vi "test-linear-system-loop-02.vi"() -> (3 "TEst Passed":bool)   [LabVIEW 2019]
uses:
  <vilib>/Rock Robotics/WPI/ThirdParty/JAS_Junk/TrajLib/LINEAR_SYSTEM_LOOP.ctl
  <vilib>/Rock Robotics/WPI/ThirdParty/JAS_Junk/TrajLib/LINEAR_QUADRATIC_REGULATOR.ctl
  <vilib>/Analysis/Matrix/Datatypes/RealMatrix.ctl
  <vilib>/Rock Robotics/WPI/ThirdParty/JAS_Junk/TrajLib/LINEAR_PLANT_INV_FF.ctl
  <vilib>/Rock Robotics/WPI/ThirdParty/JAS_Junk/TrajLib/KALMAN_FILTER.ctl
  <vilib>/Rock Robotics/WPI/ThirdParty/JAS_Junk/TrajLib/LINEAR_SYSTEM.ctl
  <vilib>/Rock Robotics/WPI/ThirdParty/JAS_Junk/TrajLib/DCMOTOR_TYPES_ENUM.ctl
  <vilib>/Rock Robotics/WPI/ThirdParty/JAS_Junk/TrajLib/MatBuilder_Create.vi
  <vilib>/Rock Robotics/WPI/ThirdParty/JAS_Junk/TrajLib/DCMotor_GetCIM.vi
  <vilib>/Rock Robotics/WPI/ThirdParty/JAS_Junk/TrajLib/DCMotor_GetAndymark9015.vi
  <vilib>/Rock Robotics/WPI/ThirdParty/JAS_Junk/TrajLib/DCMotor_GetAndymarkRs775_125.vi
  <vilib>/Rock Robotics/WPI/ThirdParty/JAS_Junk/TrajLib/DCMotor_GetBag.vi
  <vilib>/Rock Robotics/WPI/ThirdParty/JAS_Junk/TrajLib/DCMotor_GetBanebotsRs550.vi
  <vilib>/Rock Robotics/WPI/ThirdParty/JAS_Junk/TrajLib/DCMotor_GetBanebotsRs775.vi
  <vilib>/Rock Robotics/WPI/ThirdParty/JAS_Junk/TrajLib/DCMotor_GetFalcon500.vi
  <vilib>/Rock Robotics/WPI/ThirdParty/JAS_Junk/TrajLib/DCMotor_GetMiniCIM.vi
  <vilib>/Rock Robotics/WPI/ThirdParty/JAS_Junk/TrajLib/DCMotor_GetNEO.vi
  <vilib>/Rock Robotics/WPI/ThirdParty/JAS_Junk/TrajLib/DCMotor_GetNEO550.vi
  <vilib>/Rock Robotics/WPI/ThirdParty/JAS_Junk/TrajLib/DCMotor_GetRomiBuiltIn.vi
  <vilib>/Rock Robotics/WPI/ThirdParty/JAS_Junk/TrajLib/DCMotor_GetVex775Pro.vi
  <vilib>/Rock Robotics/WPI/ThirdParty/JAS_Junk/TrajLib/LinearSystem_New.vi
  <vilib>/Rock Robotics/WPI/ThirdParty/JAS_Junk/TrajLib/MatrixHelper_Zero.vi
  <vilib>/Rock Robotics/WPI/ThirdParty/JAS_Junk/TrajLib/MatBuilder_Fill.vi
  <vilib>/Rock Robotics/WPI/ThirdParty/JAS_Junk/TrajLib/Matrix_Ident.vi
  <vilib>/Analysis/baseanly.llb/A x B.vi
  <vilib>/Analysis/baseanly.llb/Real A x B.vi
  <vilib>/Rock Robotics/WPI/ThirdParty/JAS_Junk/TrajLib/MatrixHelper_CoerceSize.vi
  <vilib>/Rock Robotics/WPI/ThirdParty/JAS_Junk/TrajLib/DCMotor_New.vi
  <vilib>/Rock Robotics/WPI/ThirdParty/JAS_Junk/TrajLib/Units_RotationsPerMinuteToRadiansPerSecond.vi
  <vilib>/Analysis/7linalg.llb/Create Special Matrix.vi
  <vilib>/Analysis/7linalg.llb/Create Special Real Matrix.vi
  <vilib>/Analysis/Matrix/Numeric/Add/Add - RM,RM.vi
  <vilib>/Rock Robotics/WPI/ThirdParty/JAS_Junk/TrajLib/Trajectory_Library.lvlib
  <vilib>/ptbypt/NI_PtbyPt.lvlib
  <vilib>/Analysis/Matrix/NI_Matrix.lvlib
panel:
  out "PredictError":bool
  out "CorrectError":bool
  out "CalcYErr":bool
  out "Waveform Graph":dbl[][](graph)
  out "Issue":bool
  out "out Linear System Loop":T1
  out "LinSysLoopErr":bool
  out "LQRError":bool
  out "KalmanError":errorcluster
  out "Elev Sstem Err":bool
  # "<States,1>"
  # "<FUTURE --- CLAMP TYPE -- For now\nuse Normalize>"
  # "Steady State Gain  \n<States,Outputs>"
  # "State Estimate <Statess,1>"
  # "<States,States>"
  # "<States,Inputs>"
  # "<Outputs,States>"
  # "<Outputs,Inputs>"
  # "<States,1>"
  # "<Inputs,1>"
  # "<States,Inputs>"
  # "<States,States>"
  # "Ref State <States,1>"
  # "Comp and capped \noutput <Inputs,1>"
  # "Controller gain\n<Inputs,States>"
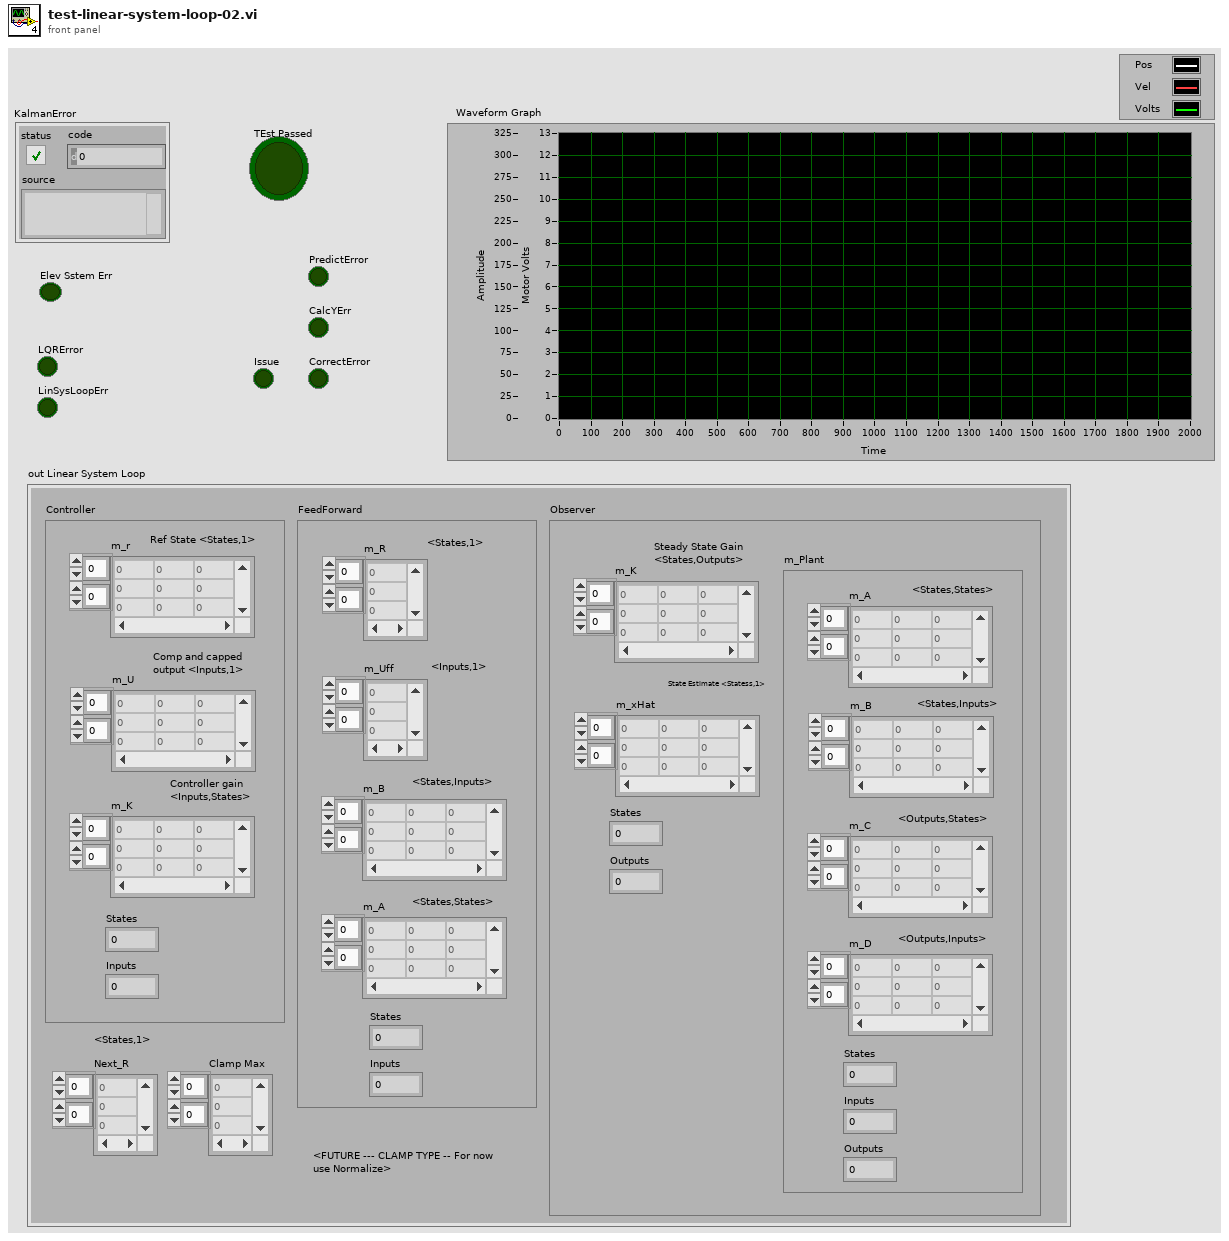
[diagram p1: front panel]
types:
  T1 = typedef "Trajectory_Library.lvlib/LINEAR_SYSTEM_LOOP.ctl" = cluster{"Controller":T2, "FeedForward":T4, "Observer":T5, "Next_R":T3, "Clamp Max":T3}
  T2 = typedef "Trajectory_Library.lvlib/LINEAR_QUADRATIC_REGULATOR.ctl" = cluster{"m_r":T3, "m_U":T3, "m_K":T3, "States":i32, "Inputs":i32}
  T3 = typedef "NI_Matrix.lvlib/RealMatrix.ctl" = dbl[][]
  T4 = typedef "Trajectory_Library.lvlib/LINEAR_PLANT_INV_FF.ctl" = cluster{"m_R":T3, "m_Uff":T3, "m_B":T3, "m_A":T3, "States":i32, "Inputs":i32}
  T5 = typedef "Trajectory_Library.lvlib/KALMAN_FILTER.ctl" = cluster{"m_K":T3, "m_xHat":T3, "States":i32, "Outputs":i32, "m_Plant":T6}
  T6 = typedef "Trajectory_Library.lvlib/LINEAR_SYSTEM.ctl" = cluster{"m_A":T3, "m_B":T3, "m_C":T3, "m_D":T3, "States":i32, "Inputs":i32, "Outputs":i32}
  T7 = typedef "Trajectory_Library.lvlib/DCMOTOR_TYPES_ENUM.ctl" = enum16{"CIM", "AndyMark 9015", "Andy Mark RS 775 125", "Bag", "BaneBots RS 550", "BaneBots RS 775", "Falcon 500", "Mini CIM", "NEO", "NEO 550", "Romi BuiltIn", "Vex 775 Pro"}
  T8 = typedef "Trajectory_Library.lvlib/DCMOTOR.CTL" = cluster{"nominalVoltage_Volts":dbl, "StallTorque_NM":dbl, "StallCurrent_Amps":dbl, "FreeCurrent_Amps":dbl, "FreeSpeed_RadPerSec":dbl, "R_Ohms":dbl, "KvINV_RadPerSecPerVolt":dbl, "Kt_NMPerAmp":dbl, "L_H":dbl, "Jr_KgM2":dbl}
  T9 = typedef "Trajectory_Library.lvlib/TRAPEZOID_PROFILE_CONSTRAINT.ctl" = cluster{"MaxVelocity":dbl, "MaxAcceleration":dbl}
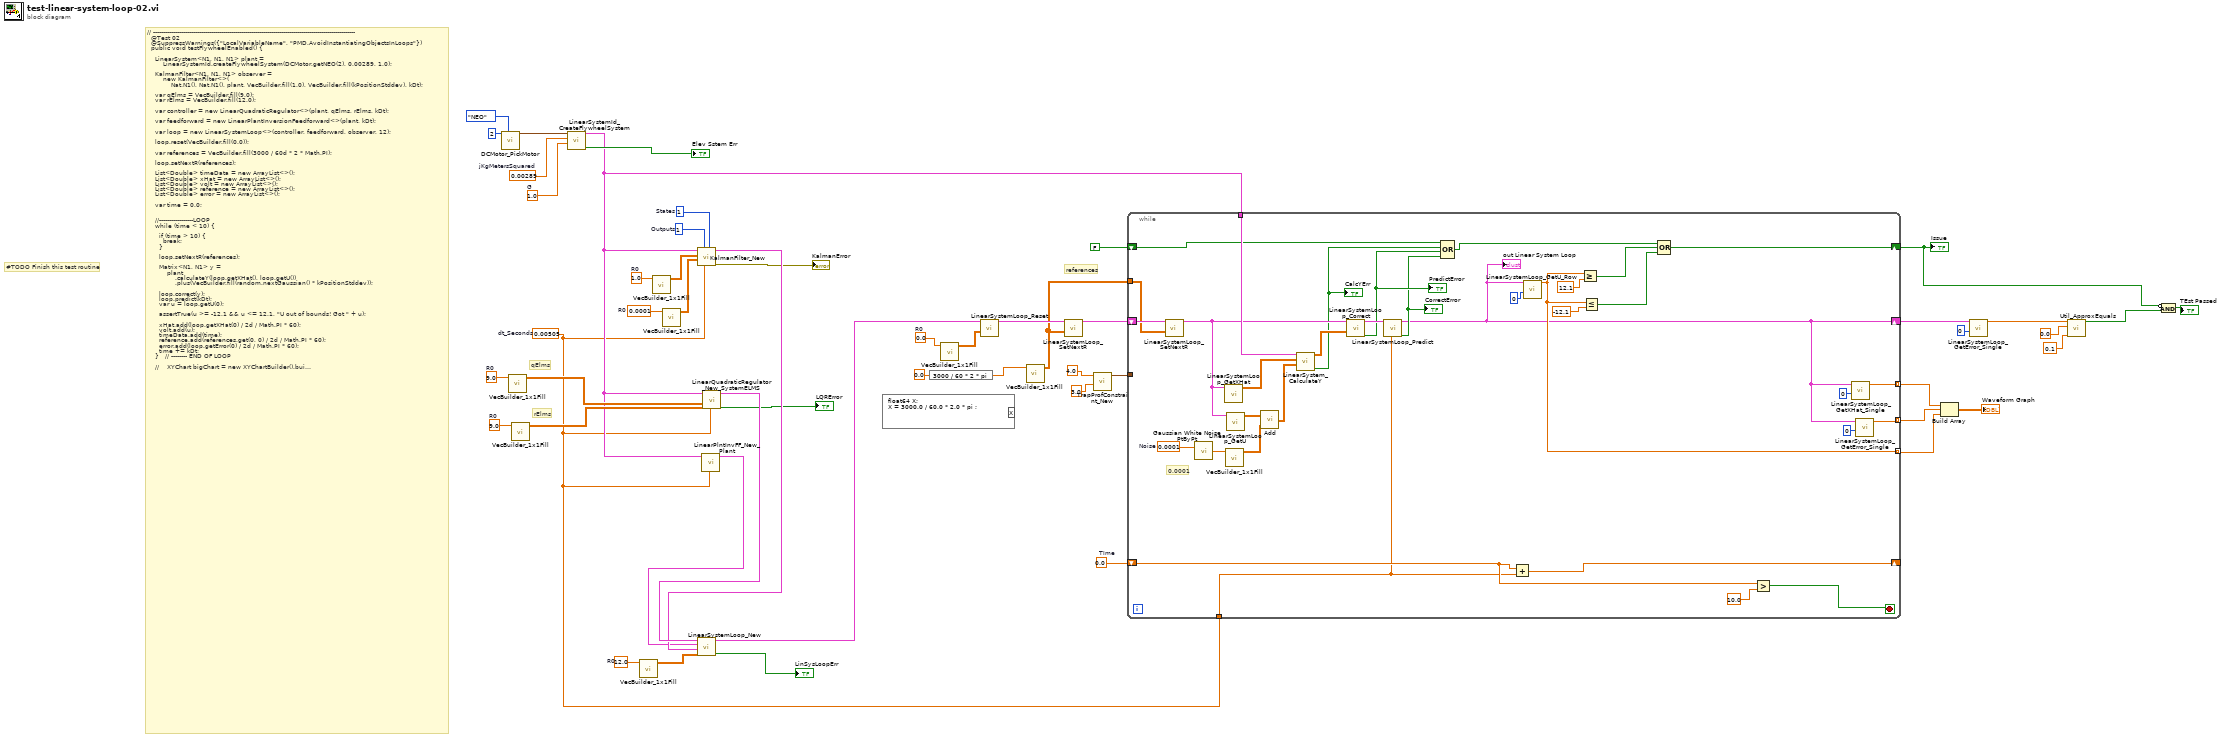
[diagram p0: block diagram]
diagram:
  w6 = 0.0  # TIme
  w10 = 12.0  # R0
  w16 = 9.0  # R0
  w17 = 9.0  # R0
  w18 = 0.00289  # jKgMetersSquared
  w36 = 0.0  # R0
  w44 = 0.0001  # R0
  w45 = 1.0  # R0
  w46 = 1  # Outputs
  w12 = 0.00505  # dt_Seconds
  w47 = 1  # States
  w51 = 1.0  # G
  # "references"
  # "rElms"
  # "qElms"
  # "#TODO Finish this test routine"
  # "// -----------------------------------------------------------------------------------------------------\n  @Test 02\n  @SuppressWarnings({\"LocalVariableName\", \"PMD.AvoidInstantiatingObjectsInLoops\"})\n  public void testFlywheelEnabled() {\n\n    LinearSystem<N1, N1, N1> plant =\n        LinearSystemId.createFlywheelSystem(DCMotor.getNEO(2), 0.00289, 1.0);\n\n    KalmanFilter<N1, N1, N1> observer =\n        new KalmanFilter<>(\n            Nat.N1(), Nat.N1(), plant, VecBuilder.fill(1.0), VecBuilder.fill(kPositionStddev), kDt);\n\n    var qElms = VecBuilder.fill(9.0);\n    var rElms = VecBuilder.fill(12.0);\n\n    var controller = new LinearQuadraticRegulator<>(plant, qElms, rElms, kDt);\n\n    var feedforward = new LinearPlantInversionFeedforward<>(plant, kDt);\n\n    var loop = new LinearSystemLoop<>(controller, feedforward, observer, 12);\n\n    loop.reset(VecBuilder.fill(0.0));\n\n    var references = VecBuilder.fill(3000 / 60d * 2 * Math.PI);\n\n    loop.setNextR(references);\n\n    List<Double> timeData = new ArrayList<>();\n    List<Double> xHat = new ArrayList<>();\n    List<Double> volt = new ArrayList<>();\n    List<Double> reference = new ArrayList<>();\n    List<Double> error = new ArrayList<>();\n\n    var time = 0.0;\n\n\n    //-----------------LOOP\n    while (time < 10) {\n\n      if (time > 10) {\n        break;\n      }\n\n      loop.setNextR(references);\n\n      Matrix<N1, N1> y =\n          plant\n              .calculateY(loop.getXHat(), loop.getU())\n              .plus(VecBuilder.fill(random.nextGaussian() * kPositionStddev));\n\n      loop.correct(y);\n      loop.predict(kDt);\n      var u = loop.getU(0);\n\n      assertTrue(u >= -12.1 && u <= 12.1, \"U out of bounds! Got \" + u);\n\n      xHat.add(loop.getXHat(0) / 2d / Math.PI * 60);\n      volt.add(u);\n      timeData.add(time);\n      reference.add(references.get(0, 0) / 2d / Math.PI * 60);\n      error.add(loop.getError(0) / 2d / Math.PI * 60);\n      time += kDt;\n    }   // -------- END OF LOOP\n\n    //    XYChart bigChart = new XYChartBuilder().build();\n    //    bigChart.addSeries(\"Xhat, RPM\", timeData, xHat);\n    //    bigChart.addSeries(\"Reference, RPM\", timeData, reference);\n    //    bigChart.addSeries(\"Error, RPM\", timeData, error);\n\n    //    XYChart smolChart = new XYChartBuilder().build();\n    //    smolChart.addSeries(\"Volts, V\", timeData, volt);\n\n    //  try {\n    //      new SwingWrapper<>(List.of(bigChart, smolChart)).displayChartMatrix();\n    //      Thread.sleep(10000000);\n    //    } catch (InterruptedException e) { e.printStackTrace(); }\n\n    assertEquals(0.0, loop.getError(0), 0.1);\n  }\n}"
  n1 = call <vilib>:"DCMotor_PickMotor.vi"("DCMOTOR_TYPES"=DCMOTOR_TYPES_ENUM."NEO", "Num Motors"=2) -> ("DCMOTOR"=w48:T8)  [unwired: 9 in]
  n2 = call <vilib>:"VecBuilder_1x1Fill.vi"("R0_C0"=w17) -> ("output matrix"=w15:T3)  [unwired: 10 in]
  n3 = call <vilib>:"VecBuilder_1x1Fill.vi"("R0_C0"=w16) -> ("output matrix"=w14:T3)  [unwired: 10 in]
  n4 = call <vilib>:"LinearSystemId_CreateFlywheelSystem.vi"("G"=w51, "jKgMetersSquared"=w18, "DCMOTOR"=w48) -> ("Error"=→"Elev Sstem Err":bool, "Linearsystem"=w13:T6)  [unwired: 7 in]
  n5 = call <vilib>:"VecBuilder_1x1Fill.vi"("R0_C0"=w10) -> ("output matrix"=w9:T3)  [unwired: 10 in]
  n6 = call <vilib>:"VecBuilder_1x1Fill.vi"("R0_C0"=w45) -> ("output matrix"=w43:T3)  [unwired: 10 in]
  n7 = call <vilib>:"VecBuilder_1x1Fill.vi"("R0_C0"=w44) -> ("output matrix"=w31:T3)  [unwired: 10 in]
  n8 = call <vilib>:"KalmanFilter_New.vi"("States"=w47, "dt_Seconds"=w12, "Outputs"=w46, "MeasurementStdDevs"=w31, "StateStdDevs"=w43, "Plant"=w13) -> ("Error"=→"KalmanError":errorcluster, "KalmanFilter"=w41:T5)  [unwired: 4 in]
  n9 = call <vilib>:"LinearPlntInvFF_New_Plant.vi"("dT_Seconds"=w12, "Plant"=w13) -> ("Linear Plnt Inversion FF"=w11:T4)  [unwired: 8 in, 1 out]
  n10 = call <vilib>:"LinearQuadraticRegulator_New_SystemELMS.vi"("dt_Seconds"=w12, "Relms"=w14, "Qelms"=w15, "LINEARSYSTEM"=w13) -> ("Error"=→"LQRError":bool, "LinearQuadraticRegulator"=w42:T2)  [unwired: 6 in]
  n11 = call <vilib>:"LinearSystemLoop_New.vi"("Max Input"=w9, "Observer"=w41, "FeedForward"=w11, "Controller"=w42) -> ("Error"=→"LinSysLoopErr":bool, "Linear System Loop"=w35:T1)  [unwired: 6 in]
  n12 = formula code="float64 X;\nX = 3000.0 / 60.0 * 2.0 * pi ;"() -> ()  [unwired: 1 out]
  n13 = expression code="3000 / 60 * 2 * pi"(0.0) -> (w7:dbl)
  n14 = call <vilib>:"VecBuilder_1x1Fill.vi"("R0_C0"=w36) -> ("output matrix"=w34:T3)  [unwired: 10 in]
  n15 = call <vilib>:"LinearSystemLoop_Reset.vi"("initialState"=w34, "input inear System Loop"=w35) -> ("out Linear System Loop"=w33:T1)  [unwired: 8 in, 1 out]
  n16 = call <vilib>:"VecBuilder_1x1Fill.vi"("R0_C0"=w7) -> ("output matrix"=w5:T3)  [unwired: 10 in]
  n17 = call <vilib>:"LinearSystemLoop_SetNextR.vi"("R"=w5, "input inear System Loop"=w33) -> ("out Linear System Loop"=w32:T1)  [unwired: 8 in, 1 out]
  n18 = call <vilib>:"TrapProfConstraint_New.vi"("Max Accel"=3.0, "Max Speed (M/S)"=4.0) -> ("TRAPEZOID_PROFILE_CONSTRAINT"=w28:T9)  [unwired: 9 in]
  n19 = while {
    tunnel: w13 -> [w66]
    tunnel: w12 -> [w61]
    shift-right: [w54] -> w3
    shift-left: w32 -> [w85]
    tunnel: w28 -> [_]
    shift-right: [w78] -> w21
    shift-left: FALSE -> [w60]
    tunnel: [w76] -> w24 mode=indexing
    tunnel: [w53] -> w23 mode=indexing
    shift-right: [w74] -> _
    shift-left: w6 -> [w75]
    tunnel: w5 -> [w71]
    tunnel: [w55] -> w4 mode=indexing
    stop <- w72 stop-if-true
    w84 = 0.0001  # Noise
    # "0.0001"
    n20 = call <vilib>:"LinearSystemLoop_SetNextR.vi"("R"=w71, "input inear System Loop"=w85) -> ("out Linear System Loop"=w64:T1)  [unwired: 8 in, 1 out]
    n21 = call <vilib>:"Gaussian White Noise PtByPt.vi"("standard deviation"=w84) -> ("Gaussian white noise"=w65:dbl)  [unwired: 2 in]
    n22 = call <vilib>:"LinearSystemLoop_GetXHat.vi"("input inear System Loop"=w64) -> ("XHat"=w67:T3)  [unwired: 10 in]
    n23 = call <vilib>:"VecBuilder_1x1Fill.vi"("R0_C0"=w65) -> ("output matrix"=w69:T3)  [unwired: 10 in]
    n24 = call <vilib>:"LinearSystemLoop_GetU.vi"("input inear System Loop"=w64) -> ("U"=w68:T3)  [unwired: 10 in]
    n25 = call-poly <vilib>:"Add.vi"("Real Matrix B"=w69, "Real Matrix A"=w68) -> ("A + B"=w70:T3)
    n26 = call <vilib>:"LinearSystem_CalculateY.vi"("ClampedU"=w70, "X"=w67, "Linearsystem"=w66) -> ("Error"=w58:bool, "outY"=w63:T3)  [unwired: 7 in]
    "CalcYErr" <- w58
    n27 = call <vilib>:"LinearSystemLoop_Correct.vi"("Y"=w63, "input inear System Loop"=w64) -> ("Error"=w57:bool, "out Linear System Loop"=w62:T1)  [unwired: 8 in]
    "PredictError" <- w57
    n28 = call <vilib>:"LinearSystemLoop_Predict.vi"("dT_Seconds"=w61, "input inear System Loop"=w62) -> ("Error"=w56:bool, "out Linear System Loop"=w54:T1)  [unwired: 8 in]
    "out Linear System Loop" <- w54
    "CorrectError" <- w56
    n29 = Compound Arithmetic op=OR(w60, w58, w57, w56) -> (w59:bool)
    n30 = Add(x=w75, y=w61) -> (x+y=w74:dbl)
    n31 = call <vilib>:"LinearSystemLoop_GetU_Row.vi"("Row"=0, "input inear System Loop"=w54) -> ("U"=w55:dbl)  [unwired: 9 in]
    n32 = Greater Or Equal?(x=w55, y=12.1) -> (x >= y?=w79:bool)
    n33 = Less Or Equal?(x=w55, y=-12.1) -> (x <= y?=w80:bool)
    n34 = Compound Arithmetic op=OR(w59, w79, w80) -> (w78:bool)
    n35 = Greater?(x=w75, y=10.0) -> (0:w72:bool)
    n36 = call <vilib>:"LinearSystemLoop_GetXHat_Single.vi"("Row"=0, "input inear System Loop"=w54) -> ("XHat"=w76:dbl)  [unwired: 9 in]
    n37 = call <vilib>:"LinearSystemLoop_GetError_Single.vi"("Row"=0, "input inear System Loop"=w54) -> ("Error"=w53:dbl)  [unwired: 9 in]
  }
  "Issue" <- w21
  n38 = Build Array(w24, w23, w4) -> (→"Waveform Graph":dbl[][])
  n39 = call <vilib>:"LinearSystemLoop_GetError_Single.vi"("Row"=0, "input inear System Loop"=w3) -> ("Error"=w1:dbl)  [unwired: 9 in]
  n40 = call <vilib>:"Util_ApproxEquals.vi"("Tolerance"=0.1, "Value 2"=0.0, "Value 1"=w1) -> ("ApproxEquals"=w20:bool)  [unwired: 8 in]
  n41 = Compound Arithmetic op=AND(invert w21, w20) -> (→"TEst Passed":bool)
